vi "OptionCycle.vi"(4 "ValuetoSet":i32, 6 "SetValue":bool, 8 "MinValue":i32, 9 "MaxValue":i32, 10 "BackwardsInput":bool, 11 "ForwardInput":bool) -> (3 "CycleNum":i32)   [LabVIEW 2020]
doc: "Cycles through a series of integer values based on a boolean input to either incremet or decrement the value. To obtain a single cycle input, recommend using \"EdgeOn.vi\" to detect whena button is pressed. \n\nInputs:\n-- ForwardInput -- Boolean -- Send a true value to increment the series by 1 --\n-- BackwardsInput -- Boolean -- Send a true value to decrement the series by 1 --\n-- MaxValue -- Integer -- The maximum value of the series (Inclusive) --\n-- MinValue -- Double -- The minimum value of the series (Exclusive) --\n\nOutputs:\n-- CycleNum -- Integer -- The current location in the series --"
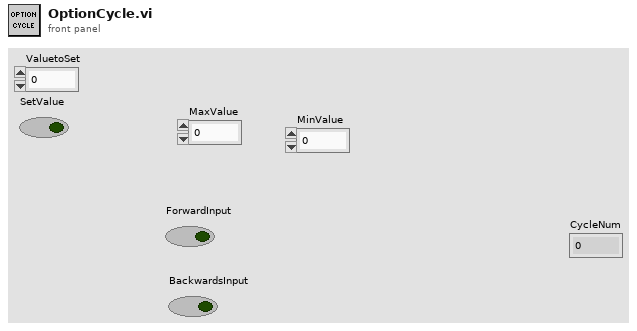
[diagram p1: front panel]
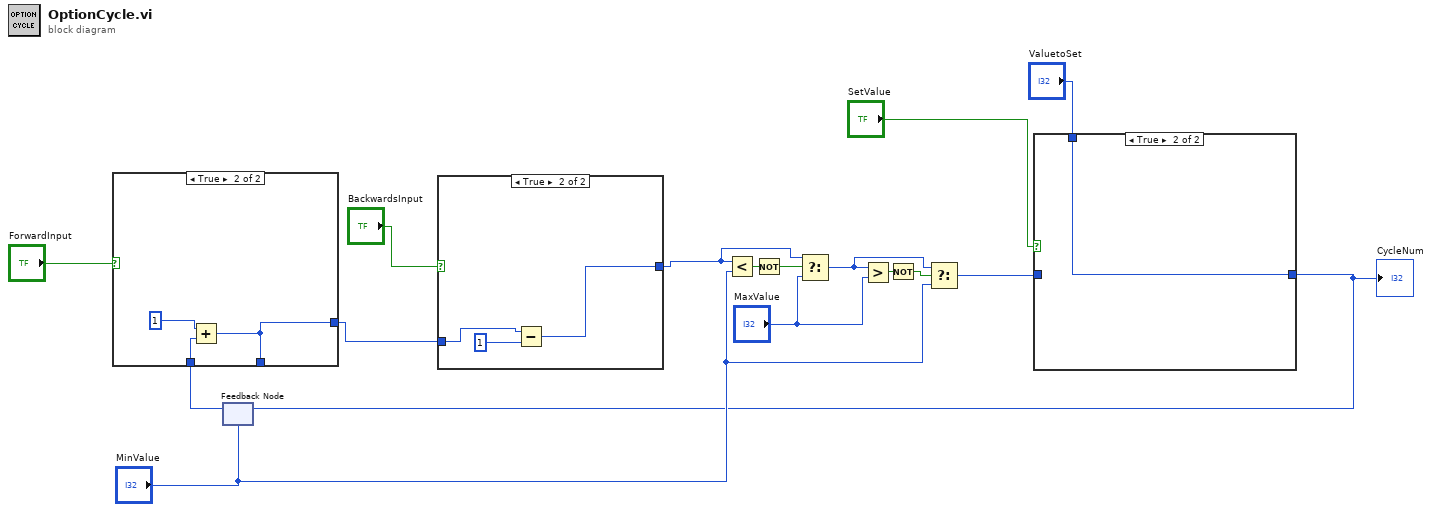
[diagram p0: block diagram]
diagram:
  n1 = feedback #1("MinValue") -> (w15:i32)
  n2 = case shown="True" "ForwardInput" {
    tunnel: [w17 w18] -> _
    tunnel: w15 -> [w17 w19]
    tunnel: [w17 w18] -> w13
    frame False {
    }
    frame True {
      n3 = Add(x=1, y=w19) -> (x+y=w18:i32)
    }
  }
  n4 = case shown="True" "BackwardsInput" {
    tunnel: [w21 w24] -> w10
    tunnel: w13 -> [w21 w22]
    frame False {
    }
    frame True {
      n5 = Subtract(x=w22, y=1) -> (x-y=w24:i32)
    }
  }
  n6 = Less?(x=w10, y="MinValue") -> (x < y?=w12:bool)
  n7 = Not(x=w12) -> (.not. x?=w11:bool)
  n8 = Select(t=w10, s=w11, f="MaxValue") -> (s? t:f=w7:i32)
  n9 = Greater?(x=w7, y="MaxValue") -> (0:w9:bool)
  n10 = Not(x=w9) -> (.not. x?=w8:bool)
  n11 = Select(t=w7, s=w8, f="MinValue") -> (s? t:f=w3:i32)
  n12 = case shown="True" "SetValue" {
    tunnel: [w25 w26] -> w4
    tunnel: w3 -> [w25 _]
    tunnel: "ValuetoSet" -> [_ w26]
    frame False {
    }
    frame True {
    }
  }
  "CycleNum" <- w4
  n13 = feedback-in #1(w4) -> ()
